vi "onDestroy.vi"(8 "error in (no error)":errorcluster, 11 "SMO.Dictionary.Variant":refnum<class "SMO.Dictionary.Variant.lvclass">) -> (0 "error out":errorcluster, 3 "SMO.Dictionary.Variant out":refnum<class "SMO.Dictionary.Variant.lvclass">)   [LabVIEW 2013, in "SMO.Dictionary.lvlib" / "SMO.Dictionary.Variant.lvclass"]
doc: "JKI State Machine Objects (SMO) 1.0.1.12\nJKI - JKI\nCopyright (c) 2016, JKI"
uses:
  SMO.Dictionary.Variant.lvclass
  SMO.Dictionary/SMO.Dictionary.lvclass
  SMO.Dictionary.Variant.lvclass/SMO.Dictionary.Variant.ctl
panel:
  # "For instructions on how to use the JKI State Machine Objects, examples and video tutorials, visit:\nhttp://jki.net/state-machine-objects/\n\nJKI State Machine Objects™\nhttp://jki.net/state-machine-objects/\nCopyright (C) 2005-2015, JKI <info@jki.net>\nALL RIGHTS RESERVED"
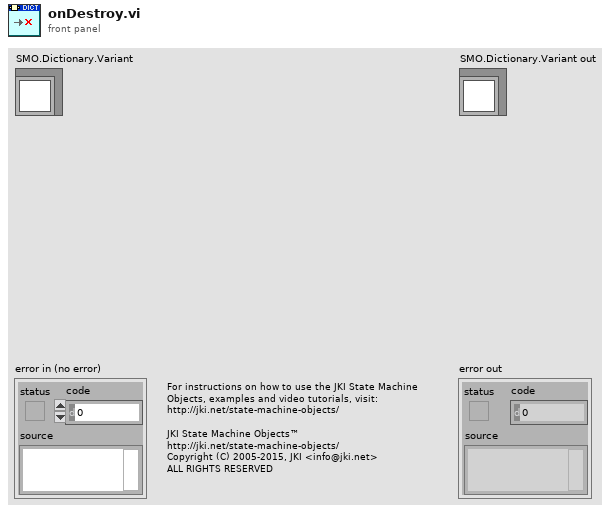
[diagram p1: front panel]
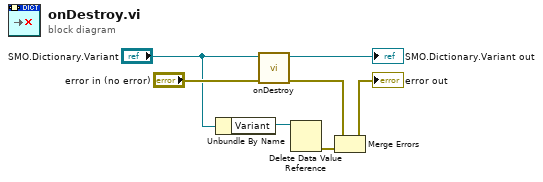
[diagram p0: block diagram]
diagram:
  n1 = Unbundle By Name("SMO.Dictionary.Variant") -> ("Variant"=w4:refnum<data-value>)
  n2 = call-parent "onDestroy.vi"("error in (no error)"="error in (no error)", "SMO"="SMO.Dictionary.Variant") -> ("error out"=w2:errorcluster, "SMO out"=→"SMO.Dictionary.Variant out":refnum<class "SMO.Dictionary.Variant.lvclass">)  [unwired: 8 in]
  n3 = Delete Data Value Reference(data value reference=w4) -> (error out=w3:errorcluster)  [unwired: 1 in, 1 out]
  n4 = Merge Errors(w2, w3) -> (→"error out":errorcluster)
